vi "单个流程校验.vi"(8 "error in (no error)":errorcluster, 10 "添加的路径":path, 11 "参数簇":T1={"启动参数"=1, "启动模式"=enum."跨度核查", "量程"=enum."低量程"} {"启动参数" items=["总磷"=1, "总氮"=2, "氨氮"=3]}) -> (0 "error out":errorcluster, 2 "结果字符串":string, 3 "check？":bool)   [LabVIEW 2016, in "斯坦道总氮V2.lvlib"]
uses:
  <vilib>/Plasmionique/MB Master/MB Master.lvlib
panel:
  out "流程":u16[](array[numeric]) format="%04xH"
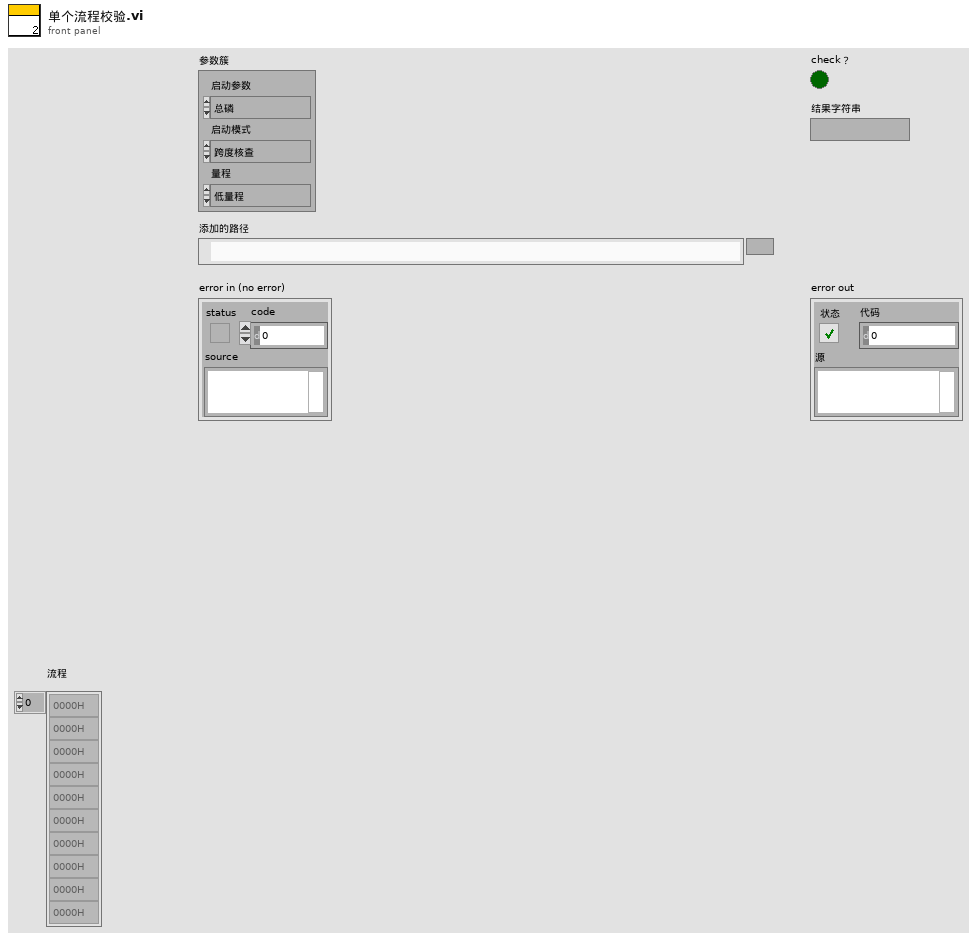
[diagram p1: front panel]
types:
  T1 = cluster{"启动参数":u16, "启动模式":enum16{"跨度核查", "水样测量", "零点核查", "标样核查", "加标回收", "快捷测试", "空白校准", "标样校准"}, "量程":enum16{"低量程", "高量程"}}
  T2 = enum16{"跨度核查", "水样测量", "零点核查", "标样核查", "加标回收", "快捷测试", "空白校准", "标样校准"}
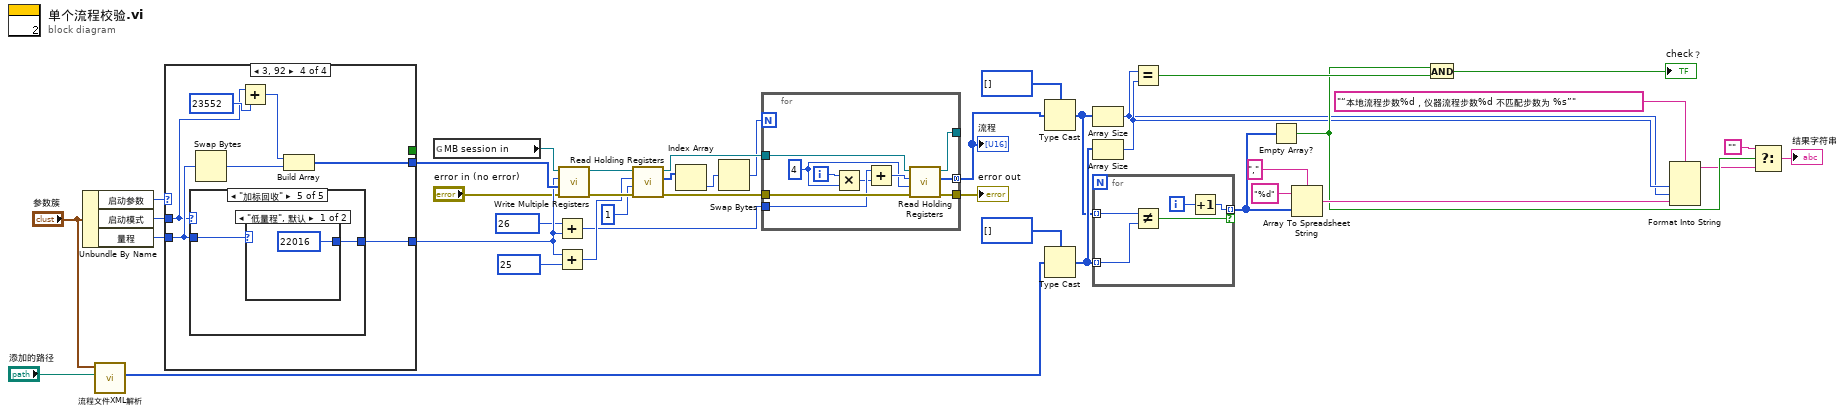
[diagram p0: block diagram]
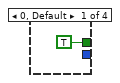
[diagram p2: hidden frame]
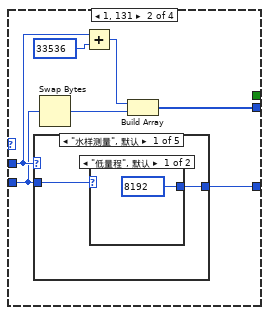
[diagram p3: hidden frame]
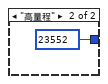
[diagram p4: hidden frame]
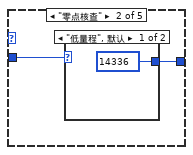
[diagram p5: hidden frame]
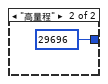
[diagram p6: hidden frame]
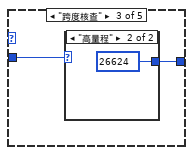
[diagram p7: hidden frame]
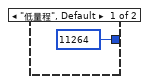
[diagram p8: hidden frame]
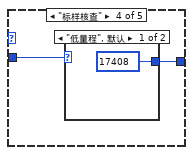
[diagram p9: hidden frame]
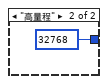
[diagram p10: hidden frame]
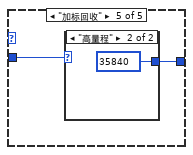
[diagram p11: hidden frame]
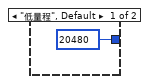
[diagram p12: hidden frame]
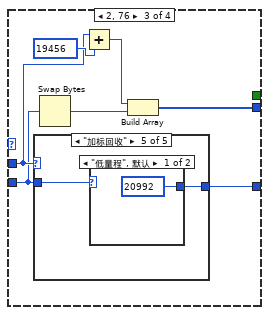
[diagram p13: hidden frame]
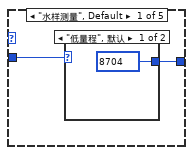
[diagram p14: hidden frame]
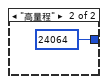
[diagram p15: hidden frame]
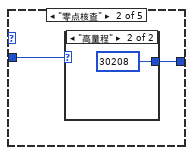
[diagram p16: hidden frame]
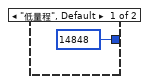
[diagram p17: hidden frame]
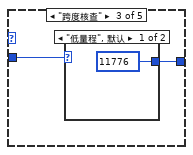
[diagram p18: hidden frame]
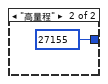
[diagram p19: hidden frame]
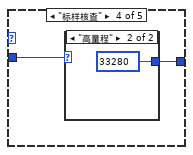
[diagram p20: hidden frame]
diagram:
  n1 = Unbundle By Name("参数簇") -> ("启动参数"=w28:u16, "启动模式"=w27:T2, "量程"=w26:enum16{"低量程", "高量程"})
  n2 = call "流程文件XML解析.vi"("添加的路径"="添加的路径", "参数簇"="参数簇") -> ("通讯数据"=w7:u16[])  [unwired: 8 in, 1 out]
  n3 = case shown="3, 92" w28 {
    tunnel: w27 -> [_ w47 w72 w98]
    tunnel: w26 -> [_ w46 w71 w99]
    tunnel: [_ w49 w76 w103] -> w32
    tunnel: [TRUE _ _ _] -> _
    tunnel: [_ w43 w70 w97] -> w39
    frame 0, Default {
    }
    frame 1, 131 {
      n4 = case shown="\"水样测量\", 默认" w47 {
        tunnel: w46 -> [w51 w55 w59 w63 w67]
        tunnel: [w50 w54 w58 w62 w66] -> w49
        frame "水样测量", Default {
          n5 = case shown="\"低量程\", 默认" w51 {
            tunnel: [u16 8192 ("starting address") u16 23552 ("starting address")] -> w50
            frame "低量程", Default {
            }
            frame "高量程" {
            }
          }
        }
        frame "零点核查" {
          n6 = case shown="\"低量程\", 默认" w55 {
            tunnel: [u16 14336 ("starting address") u16 29696 ("starting address")] -> w54
            frame "低量程", Default {
            }
            frame "高量程" {
            }
          }
        }
        frame "跨度核查" {
          n7 = case shown="\"高量程\"" w59 {
            tunnel: [u16 11264 ("starting address") u16 26624 ("starting address")] -> w58
            frame "低量程", Default {
            }
            frame "高量程" {
            }
          }
        }
        frame "标样核查" {
          n8 = case shown="\"低量程\", 默认" w63 {
            tunnel: [u16 17408 ("starting address") u16 32768 ("starting address")] -> w62
            frame "低量程", Default {
            }
            frame "高量程" {
            }
          }
        }
        frame "加标回收" {
          n9 = case shown="\"高量程\"" w67 {
            tunnel: [u16 20480 ("starting address") u16 35840 ("starting address")] -> w66
            frame "低量程", Default {
            }
            frame "高量程" {
            }
          }
        }
      }
      n10 = Swap Bytes(anything=w46) -> (byte swapped=w45:u16)
      n11 = Add(x=w47, y=u16 33536 ("starting address")) -> (x+y=w44:u16)
      n12 = Build Array(w44, w45) -> (w43:u16[])
    }
    frame 2, 76 {
      n13 = case shown="\"加标回收\"" w72 {
        tunnel: w71 -> [w78 w82 w86 w90 w94]
        tunnel: [w77 w81 w85 w89 w93] -> w76
        frame "水样测量", Default {
          n14 = case shown="\"低量程\", 默认" w78 {
            tunnel: [u16 8704 ("starting address") u16 24064 ("starting address")] -> w77
            frame "低量程", Default {
            }
            frame "高量程" {
            }
          }
        }
        frame "零点核查" {
          n15 = case shown="\"高量程\"" w82 {
            tunnel: [u16 14848 ("starting address") u16 30208 ("starting address")] -> w81
            frame "低量程", Default {
            }
            frame "高量程" {
            }
          }
        }
        frame "跨度核查" {
          n16 = case shown="\"低量程\", 默认" w86 {
            tunnel: [u16 11776 ("starting address") u16 27155 ("starting address")] -> w85
            frame "低量程", Default {
            }
            frame "高量程" {
            }
          }
        }
        frame "标样核查" {
          n17 = case shown="\"高量程\"" w90 {
            tunnel: [u16 17920 ("starting address") u16 33280 ("starting address")] -> w89
            frame "低量程", Default {
            }
            frame "高量程" {
            }
          }
        }
        frame "加标回收" {
          n18 = case shown="\"低量程\", 默认" w94 {
            tunnel: [u16 20992 ("starting address") u16 36352 ("starting address")] -> w93
            frame "低量程", Default {
            }
            frame "高量程" {
            }
          }
        }
      }
      n19 = Swap Bytes(anything=w71) -> (byte swapped=w74:u16)
      n20 = Add(x=w72, y=u16 19456 ("starting address")) -> (x+y=w73:u16)
      n21 = Build Array(w73, w74) -> (w70:u16[])
    }
    frame 3, 92 {
      n22 = case shown="\"加标回收\"" w98 {
        tunnel: w99 -> [w105 w109 w113 w117 w121]
        tunnel: [w104 w108 w112 w116 w120] -> w103
        frame "水样测量", Default {
          n23 = case shown="\"低量程\", 默认" w105 {
            tunnel: [u16 9728 ("starting address") u16 25088 ("starting address")] -> w104
            frame "低量程", Default {
            }
            frame "高量程" {
            }
          }
        }
        frame "零点核查" {
          n24 = case shown="\"低量程\", 默认" w109 {
            tunnel: [u16 15872 ("starting address") u16 31232 ("starting address")] -> w108
            frame "低量程", Default {
            }
            frame "高量程" {
            }
          }
        }
        frame "跨度核查" {
          n25 = case shown="\"低量程\", 默认" w113 {
            tunnel: [u16 12800 ("starting address") u16 28160 ("starting address")] -> w112
            frame "低量程", Default {
            }
            frame "高量程" {
            }
          }
        }
        frame "标样核查" {
          n26 = case shown="\"高量程\"" w117 {
            tunnel: [u16 18944 ("starting address") u16 34304 ("starting address")] -> w116
            frame "低量程", Default {
            }
            frame "高量程" {
            }
          }
        }
        frame "加标回收" {
          n27 = case shown="\"低量程\", 默认" w121 {
            tunnel: [u16 22016 ("starting address") u16 37376 ("starting address")] -> w120
            frame "低量程", Default {
            }
            frame "高量程" {
            }
          }
        }
      }
      n28 = Swap Bytes(anything=w99) -> (byte swapped=w101:u16)
      n29 = Add(x=w98, y=u16 23552 ("starting address")) -> (x+y=w100:u16)
      n30 = Build Array(w100, w101) -> (w97:u16[])
    }
  }
  n31 = global read "VAR总磷总氮全局变量.vi" "MB session in"() -> (w29:refnum<class "MB_Master.lvclass">)
  n32 = Add(x=u16 26 ("starting address"), y=w32) -> (x+y=w30:u16)
  n33 = Add(x=w32, y=u16 25 ("starting address")) -> (x+y=w35:u16)
  n34 = call <vilib>:"Write Multiple Registers.vi"("error in (no error)"="error in (no error)", "values"=w39, "starting address"=w32, "MB session in"=w29) -> ("error out"=w37:errorcluster, "MB session out"=w38:refnum<class "MB_Master.lvclass">)  [unwired: 6 in]
  n35 = call <vilib>:"Read Holding Registers.vi"("error in (no error)"=w37, "quantity"=u16 1, "starting address"=w35, "MB session in"=w38) -> ("error out"=w33:errorcluster, "Registers"=w22:u16[], "MB session out"=w34:refnum<class "MB_Master.lvclass">)  [unwired: 5 in]
  n36 = Index Array(array=w22) -> (element=w21:u16)  [unwired: 1 in]
  n37 = Swap Bytes(anything=w21) -> (byte swapped=w1:u16)
  n38 = for {
    N: w1 -> [_]
    tunnel: w34 -> [w133]
    tunnel: w33 -> [w132]
    tunnel: w30 -> [w131]
    tunnel: [w128] -> _
    tunnel: [w127] -> w24
    tunnel: [w124] -> w6 mode=concatenating
    i -> [w130]
    w125 = 4 ("y")
    n39 = Multiply(x=w130, y=w125) -> (x*y=w126:i32)
    n40 = Add(x=w131, y=w126) -> (x+y=w129:i32)
    n41 = call <vilib>:"Read Holding Registers.vi"("error in (no error)"=w132, "quantity"=w125, "starting address"=w129, "MB session in"=w133) -> ("error out"=w127:errorcluster, "Registers"=w124:u16[], "MB session out"=w128:refnum<class "MB_Master.lvclass">)  [unwired: 5 in]
  }
  "error out" <- w24
  "流程" <- w6
  n42 = Type Cast(type=u64[] [], x=w6) -> (*(type *) &x=w3:u64[])
  n43 = Type Cast(type=u64[] [], x=w7) -> (*(type *) &x=w5:u64[])
  n44 = Array Size(array=w3) -> (size(s)=w2:i32)
  n45 = Array Size(array=w5) -> (size(s)=w4:i32)
  n46 = for {
    tunnel: w3 -> [w137] mode=indexing
    tunnel: w5 -> [w138] mode=indexing
    tunnel: [w134] -> w8 mode=indexing if=w136
    i -> [w135]
    n47 = Not Equal?(x=w137, y=w138) -> (x != y?=w136:bool)
    n48 = Increment(x=w135) -> (x+1=w134:i32)
  }
  n49 = Equal?(x=w2, y=w4) -> (x = y?=w20:bool)
  n50 = Empty Array?(array=w8) -> (empty?=w14:bool)
  n51 = Array To Spreadsheet String(delimiter (Tab)="," ("分隔符(Tab)"), array=w8, 3:"%d" ("格式字符串")) -> (spreadsheet string=w15:string)
  n52 = And(x=w14, y=w20) -> (x .and. y?=→"check？":bool)
  n53 = Format Into String(format string="“本地流程步数%d，仪器流程步数%d 不匹配步数为 %s”" ("格式字符串"), w4, w2, w15) -> (resulting string=w13:string)  [unwired: 2 in, 1 out]
  n54 = Select(t="", s=w14, f=w13) -> (s? t:f=→"结果字符串":string)
